vi "writeValveSetpoints.vi"(8 "error in (no error)":errorcluster, 10 "ILC in":refnum<class "ILC.lvclass">, 11 "IActuatorCylinder in":refnum<class "ILCControlledActuatorCylinder.lvclass">) -> (0 "error out":errorcluster, 2 "ILC out":refnum<class "ILC.lvclass">, 3 "IActuatorCylinder out":refnum<class "ILCControlledActuatorCylinder.lvclass">)   [LabVIEW 2015, in "ILCControlledActuatorCylinder.lvclass"]
uses:
  ILCControlledActuatorCylinder.lvclass
  ILCDAC/IILCDAC/IILCDAC.lvclass
  Calculators/VoltageToILCDACRaw/VoltageToILCDACRaw.lvclass
  <userlib>/Common/ILC/ILC/ILC.lvclass
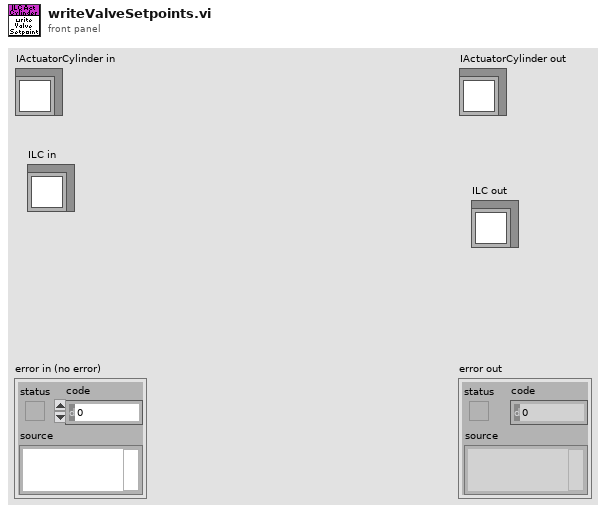
[diagram p1: front panel]
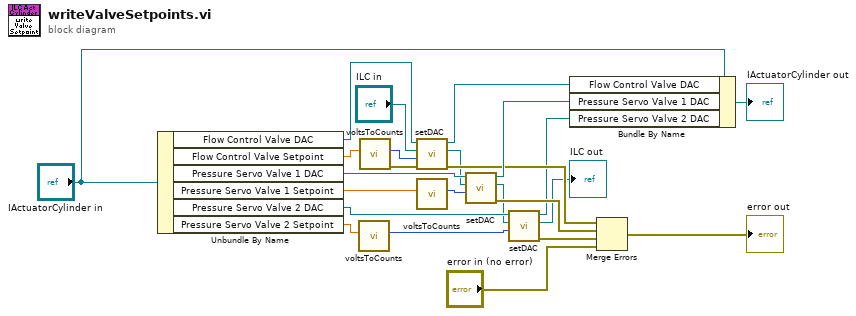
[diagram p0: block diagram]
diagram:
  n1 = Unbundle By Name("IActuatorCylinder in") -> ("Flow Control Valve DAC"=w24:refnum<class "IILCDAC.lvclass">, "Flow Control Valve Setpoint"=w9:dbl[unit], "Pressure Servo Valve 1 DAC"=w23:refnum<class "IILCDAC.lvclass">, "Pressure Servo Valve 1 Setpoint"=w8:dbl[unit], "Pressure Servo Valve 2 DAC"=w14:refnum<class "IILCDAC.lvclass">, "Pressure Servo Valve 2 Setpoint"=w11:dbl[unit])
  n2 = call "voltsToCounts.vi"("Voltage"=w11) -> ("DAC Counts"=w7:u16)  [unwired: 8 in, 2 out]
  n3 = call "voltsToCounts.vi"("Voltage"=w9) -> ("error out"=w10:errorcluster, "DAC Counts"=w5:u16)  [unwired: 8 in, 1 out]
  n4 = call-dynamic "setDAC.vi"("error in (no error)"=w10, "DAC Value"=w5, "ILC in"="ILC in", "IILCDAC in"=w24) -> ("error out"=w16:errorcluster, "ILC out"=w3:refnum<class "ILC.lvclass">, "IILCDAC out"=w20:refnum<class "IILCDAC.lvclass">)  [unwired: 5 in]
  n5 = call "voltsToCounts.vi"("Voltage"=w8) -> ("DAC Counts"=w6:u16)  [unwired: 8 in, 2 out]
  n6 = call-dynamic "setDAC.vi"("DAC Value"=w6, "ILC in"=w3, "IILCDAC in"=w23) -> ("error out"=w15:errorcluster, "ILC out"=w2:refnum<class "ILC.lvclass">, "IILCDAC out"=w19:refnum<class "IILCDAC.lvclass">)  [unwired: 6 in]
  n7 = call-dynamic "setDAC.vi"("DAC Value"=w7, "ILC in"=w2, "IILCDAC in"=w14) -> ("error out"=w12:errorcluster, "ILC out"=→"ILC out":refnum<class "ILC.lvclass">, "IILCDAC out"=w13:refnum<class "IILCDAC.lvclass">)  [unwired: 6 in]
  n8 = Bundle By Name(cluster="IActuatorCylinder in", "Flow Control Valve DAC"=w20, "Pressure Servo Valve 1 DAC"=w19, "Pressure Servo Valve 2 DAC"=w13) -> (→"IActuatorCylinder out":refnum<class "ILCControlledActuatorCylinder.lvclass">)
  n9 = Merge Errors(w16, w15, w12, "error in (no error)") -> (→"error out":errorcluster)
